vi "HopperButtonControl.vi"(4 "AutoLowerButton":bool, 5 "AutoRaiseButton":bool, 6 "ManualLowerButton":bool, 7 "ManualRaiseButton":bool) -> ()   [LabVIEW 2016, in "2039lib.lvlib"]
uses:
  Tr/2017 Master Code (Robot)/2039lib.lvlib
  HopperStates.ctl
  Tr/2017 Master Code (Robot)/Robot Global Data.vi
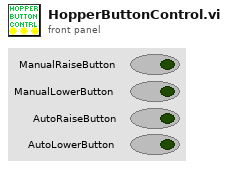
[diagram p1: front panel]
types:
  T1 = typedef "2039lib.lvlib/HopperStates.ctl" = enum16{"HopperIdle", "ManualRaiseHopper", "ManualLowerHopper", "AutoRaiseHopper", "AutoLowerHopper", "AtTop", "AtBottom"}
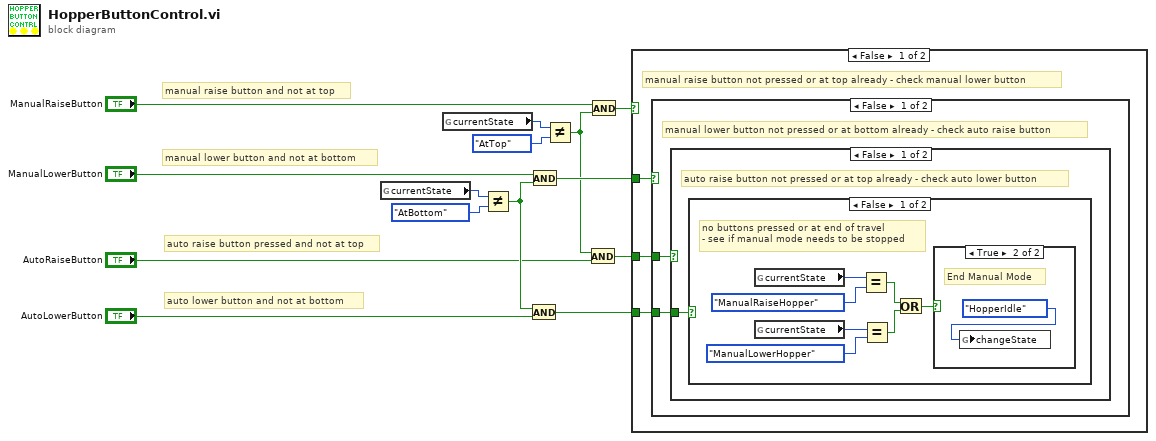
[diagram p0: block diagram]
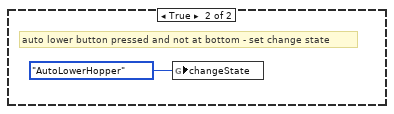
[diagram p3: hidden frame]
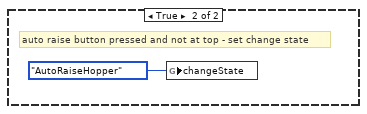
[diagram p4: hidden frame]
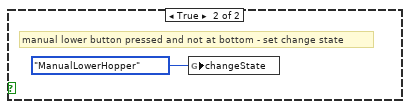
[diagram p5: hidden frame]
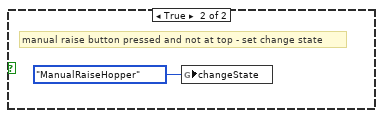
[diagram p6: hidden frame]
diagram:
  # "auto lower button and not at bottom"
  # "auto raise button pressed and not at top"
  # "manual lower button and not at bottom"
  # "manual raise button and not at top"
  n1 = global read "Robot Global Data.vi" "currentState"() -> (w6:T1)
  n2 = global read "Robot Global Data.vi" "currentState"() -> (w1:T1)
  n3 = Not Equal?(x=w6, y=HopperStates."AtBottom") -> (x != y?=w13:bool)
  n4 = And(x=w13, y="AutoLowerButton") -> (x .and. y?=w14:bool)
  n5 = And(x="ManualLowerButton", y=w13) -> (x .and. y?=w12:bool)
  n6 = Not Equal?(x=w1, y=HopperStates."AtTop") -> (x != y?=w10:bool)
  n7 = And(x=w10, y="AutoRaiseButton") -> (x .and. y?=w4:bool)
  n8 = And(x="ManualRaiseButton", y=w10) -> (x .and. y?=w3:bool)
  n9 = case shown="False" w3 {
    tunnel: w12 -> [w17 _]
    tunnel: w4 -> [w16 _]
    tunnel: w14 -> [w15 _]
    frame False {
      # "manual raise button not pressed or at top already - check manual lower button"
      n10 = case shown="False" w17 {
        tunnel: w16 -> [w19 _]
        tunnel: w15 -> [w18 _]
        frame False {
          # "manual lower button not pressed or at bottom already - check auto raise button"
          n11 = case shown="False" w19 {
            tunnel: w18 -> [w20 _]
            frame False {
              # "auto raise button not pressed or at top already - check auto lower button"
              n12 = case shown="False" w20 {
                frame False {
                  # "no buttons pressed or at end of travel \n- see if manual mode needs to be stopped"
                  n13 = global read "Robot Global Data.vi" "currentState"() -> (w27:T1)
                  n14 = global read "Robot Global Data.vi" "currentState"() -> (w25:T1)
                  n15 = Equal?(x=w27, y=HopperStates."ManualRaiseHopper" ("changeState")) -> (x = y?=w23:bool)
                  n16 = Equal?(x=w25, y=HopperStates."ManualLowerHopper" ("changeState")) -> (x = y?=w22:bool)
                  n17 = Or(x=w23, y=w22) -> (x .or. y?=w21:bool)
                  n18 = case shown="True" w21 {
                    frame False {
                      # "Not in manual mode\n- do nothing here"
                    }
                    frame True {
                      # "End Manual Mode"
                      n19 = global write "Robot Global Data.vi" "changeState"(HopperStates."HopperIdle" ("changeState")) -> ()
                    }
                  }
                }
                frame True {
                  # "auto lower button pressed and not at bottom - set change state"
                  n20 = global write "Robot Global Data.vi" "changeState"(HopperStates."AutoLowerHopper" ("changeState")) -> ()
                }
              }
            }
            frame True {
              # "auto raise button pressed and not at top - set change state"
              n21 = global write "Robot Global Data.vi" "changeState"(HopperStates."AutoRaiseHopper" ("changeState")) -> ()
            }
          }
        }
        frame True {
          # "manual lower button pressed and not at bottom - set change state"
          n22 = global write "Robot Global Data.vi" "changeState"(HopperStates."ManualLowerHopper" ("changeState")) -> ()
        }
      }
    }
    frame True {
      # "manual raise button pressed and not at top - set change state"
      n23 = global write "Robot Global Data.vi" "changeState"(HopperStates."ManualRaiseHopper" ("changeState")) -> ()
    }
  }
